vi "Create Line Object.vi"(5 "Line Style":T1, 7 "Line Width":sgl, 8 "error in (no error)":errorcluster, 9 "Antialiasing":bool, 10 "Alpha":sgl, 11 "Mesh Ref In":refnum<vi>) -> (0 "error out":errorcluster, 3 "Object Ref Out":refnum<vi>)   [LabVIEW 2020, in "3D Plot.lvclass"]
uses:
  <vilib>/Math Plots/3D Math Plots/3D Plot/3D Plot/3D Plot.lvclass
  <vilib>/Math Plots/3D Math Plots/3D Plot/3D Plot/Typedef/Line Type.ctl
  <vilib>/picture/3D Picture Control/Object/Create Object (name).vi
  <vilib>/picture/3D Picture Control/NI_3D Picture Control.lvlib
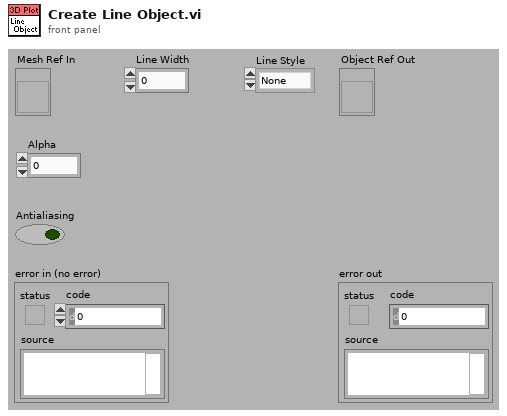
[diagram p1: front panel]
types:
  T1 = typedef "3D Plot.lvclass/Line Type.ctl" = enum16{"None", "Solid", "Dash", "Dot", "Dash Dot"}
  T2 = enum16{"Normal Bin", "Opaque Bin", "Transparent Bin"}
  T3 = enum16{"Inherit Value", "Points", "Wireframe", "Polygons"}
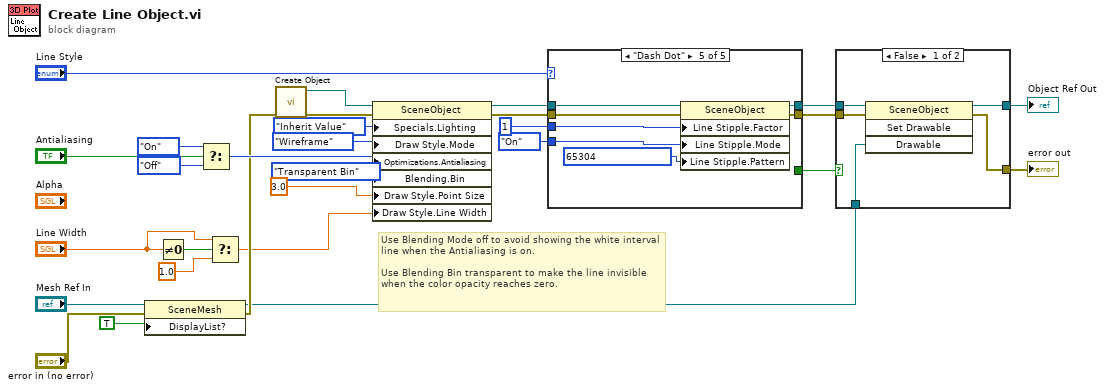
[diagram p0: block diagram]
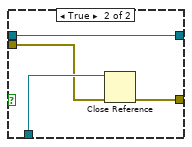
[diagram p2: hidden frame]
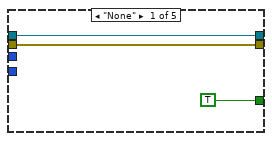
[diagram p3: hidden frame]
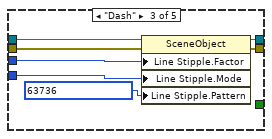
[diagram p5: hidden frame]
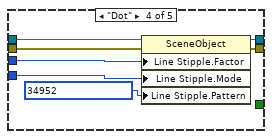
[diagram p6: hidden frame]
diagram:
  # "Use Blending Mode off to avoid showing the white interval line when the Antialiasing is on.\n\nUse Blending Bin transparent to make the line invisible when the color opacity reaches zero."
  n1 = property class="SceneMesh"(reference="Mesh Ref In", error in="error in (no error)", "DisplayList?"=TRUE ("Use Display List?")) -> (reference out=w19:refnum<vi>, error out=w22:errorcluster)
  n2 = Not Equal To 0?(x="Line Width") -> (x != 0?=w13:bool)
  n3 = Select(t=enum16{"Inherit Value", "Off", "On"}."On" ("Optimizations:Antialiasing"), s="Antialiasing", f=enum16{"Inherit Value", "Off", "On"}."Off") -> (s? t:f=w28:enum16{"Inherit Value", "Off", "On"})
  n4 = Select(t="Line Width", s=w13, f=sgl 1.0) -> (s? t:f=w10:sgl)
  n5 = call-poly <vilib>:"Create Object.vi"("error in (no error)"=w22) -> ("error out"=w23:errorcluster, "Scene:New Object"=w20:refnum<vi>)  [unwired: 9 in]
  n6 = property class="SceneObject"(reference=w20, error in=w23, "Specials.Lighting"=enum16{"Inherit Value", "Off", "On"}."Inherit Value" ("Specials:Lighting"), "Draw Style.Mode"=T3."Wireframe" ("Draw Style:Mode"), "Optimizations.Antialiasing"=w28, "Blending.Bin"=T2."Transparent Bin" ("Blending:Bin"), "Draw Style.Point Size"=sgl 3.0 ("Draw Style:Point Size"), "Draw Style.Line Width"=w10) -> (reference out=w8:refnum<vi>, error out=w7:errorcluster)
  n7 = case shown="\"Dash Dot\"" "Line Style" {
    tunnel: w8 -> [w32 w34 w41 w48 w55]
    tunnel: [w32 w34 w40 w44 w51] -> w4
    tunnel: w7 -> [w31 w33 w39 w47 w54]
    tunnel: [w31 w33 w38 w43 w50] -> w3
    tunnel: enum16{"Inherit Value", "Off", "On"}."On" ("Line Stipple:Mode") -> [_ _ w37 w45 w52]
    tunnel: 1 ("Line Stipple:Factor") -> [_ _ w36 w46 w53]
    tunnel: [TRUE _ _ _ _] -> w1
    frame "None" {
    }
    frame "Solid", Default {
    }
    frame "Dash" {
      n8 = property class="SceneObject"(reference=w41, error in=w39, "Line Stipple.Factor"=w36, "Line Stipple.Mode"=w37, "Line Stipple.Pattern"=u16 63736 ("Line Stipple:Factor")) -> (reference out=w40:refnum<vi>, error out=w38:errorcluster)
    }
    frame "Dot" {
      n9 = property class="SceneObject"(reference=w48, error in=w47, "Line Stipple.Factor"=w46, "Line Stipple.Mode"=w45, "Line Stipple.Pattern"=u16 34952 ("Line Stipple:Factor")) -> (reference out=w44:refnum<vi>, error out=w43:errorcluster)
    }
    frame "Dash Dot" {
      n10 = property class="SceneObject"(reference=w55, error in=w54, "Line Stipple.Factor"=w53, "Line Stipple.Mode"=w52, "Line Stipple.Pattern"=u16 65304 ("Line Stipple:Factor")) -> (reference out=w51:refnum<vi>, error out=w50:errorcluster)
    }
  }
  n11 = case shown="False" w1 {
    tunnel: [w60 w61] -> w29
    tunnel: [w59 w63] -> w24
    tunnel: w19 -> [w58 w64]
    tunnel: w4 -> [w57 w63]
    tunnel: w3 -> [w56 w62]
    frame False {
      n12 = invoke class="SceneObject" method="Set Drawable"(reference=w57, error in=w56, "Drawable"=w58) -> (reference out=w59:refnum<vi>, error out=w60:errorcluster)  [unwired: 1 in, 2 out]
    }
    frame True {
      n13 = Close Reference(reference=w64, error in (no error)=w62) -> (error out=w61:errorcluster)
    }
  }
  "error out" <- w29
  "Object Ref Out" <- w24
